vi "Agilent 2000 3000 X-Series Control Loop Response Analysis.vi"() -> ()   [LabVIEW 2015]
doc: "This example shows how to apply a control loop response analysis and read the analysis result."
uses:
  Agilent 2000 3000 X-Series.lvlib
  Public/Configure/Power Analysis/Configure Control Loop Response Power Analysis (Basic).vi
  Public/Data/Read Control Loop Response Power Analysis (Data).vi
  Public/Configure/Power Analysis/Configure Control Loop Response Power Analysis (Frequency).vi
  Public/Data/Read Control Loop Response Power Analysis (Gain).vi
  Public/Configure/Power Analysis/Configure Control Loop Response Power Analysis (Waveform).vi
panel:
  in  "Stop Frequency (6: 20000000 Hz)":i32(ring)=6 items=["100", "1000", "10000", "100000", "1000000", "10000000", "20000000"]
  in  "Start Frequency (1: 100 Hz)":i32(ring)=1 items=["20", "100", "1000", "10000", "100000", "1000000", "10000000"]
  out "Analysis Result":string[][](table)
  in  "Point Number (10: 10)":i32(ring)=10 items=["10"=10, "20"=20, "30"=30, "40"=40, "50"=50, "60"=60, "70"=70, "80"=80, "90"=90, "100"=100]
  in  "Amplitude (0.2)":dbl=0.2
  in  "VISA resource name":refnum<visa-resource-name>
  out "Phase Crossover Frequency (Hz)":dbl
  out "Gain Margin (dB)":dbl
  in  "Impedance (1: 50 Ohm)":i32(ring)=1 items=["1 MOhm", "50 Ohm"]
  in  "Trace (4: Gain and Phase)":i32(ring)=4 items=["None", "All", "Gain", "Phase", "Gain and Phase"]
  in  "Input Channel (0: Channel 1)":i32(ring) items=["Channel 1", "Channel 2", "Channel 3", "Channel 4"]
  in  "Output Channel (1: Channel 2)":i32(ring)=1 items=["Channel 1", "Channel 2", "Channel 3", "Channel 4"]
  # "(c) 2018 - 2023 National Instruments.  ALL RIGHTS RESERVED."
  # "Control Loop Response Analysis settings"
  # "Result"
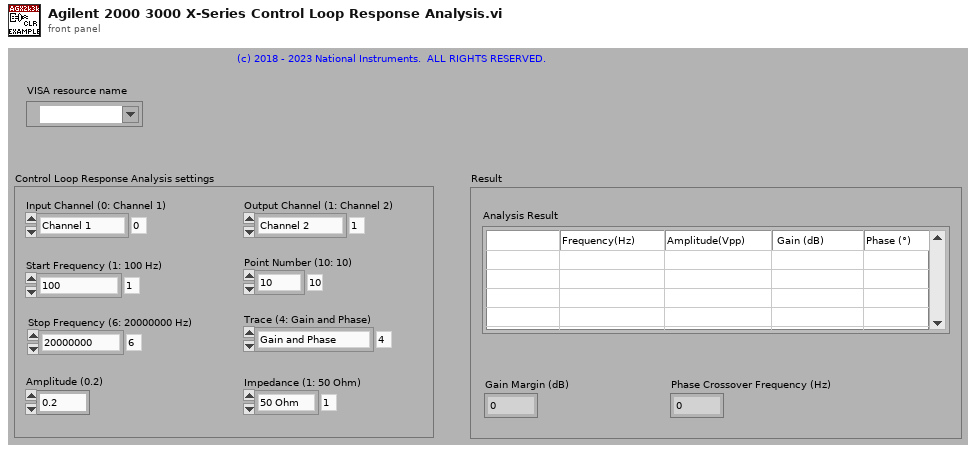
[diagram p1: front panel]
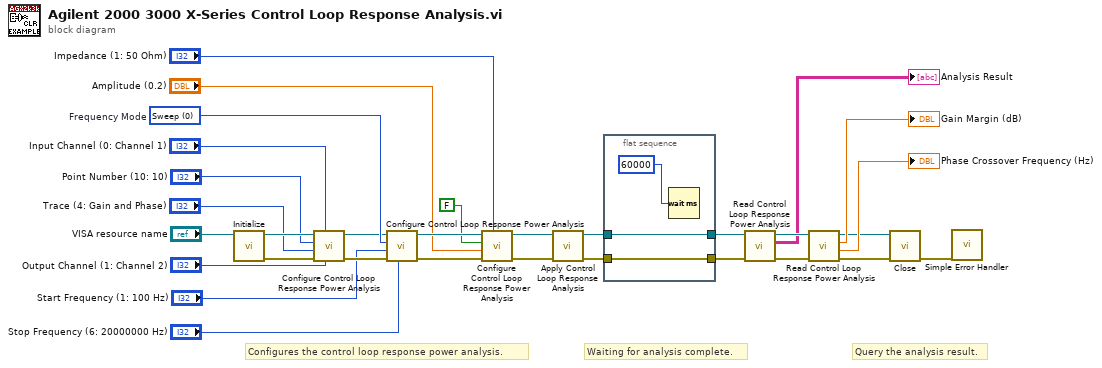
[diagram p0: block diagram]
diagram:
  w31 = 0 items=["Sweep", "Single"]  # Frequency Mode
  # "Query the analysis result."
  # "Waiting for analysis complete."
  # "Configures the control loop response power analysis."
  n1 = call "Initialize.vi"("VISA resource name"="VISA resource name") -> ("error out"=w22:errorcluster, "VISA resource name out"=w23:refnum<visa-resource-name>)  [unwired: 4 in, 5 out]
  n2 = call-poly "Configure Control Loop Response Power Analysis.vi"("Output Channel (1: Channel 2)"="Output Channel (1: Channel 2)", "Input Channel (0: Channel 1)"="Input Channel (0: Channel 1)", "error in (no error)"=w22, "Trace (4: Gain and Phase)"="Trace (4: Gain and Phase)", "Point Number (10: 10)"="Point Number (10: 10)", "VISA resource name"=w23) -> ("error out"=w19:errorcluster, "VISA resource name out"=w27:refnum<visa-resource-name>)  [unwired: 4 in]
  n3 = call-poly "Configure Control Loop Response Power Analysis.vi"("Stop Frequency (6: 20000000 Hz)"="Stop Frequency (6: 20000000 Hz)", "error in (no error)"=w19, "Start Frequency (1: 100 Hz)"="Start Frequency (1: 100 Hz)", "Frequency Mode (0: Sweep)"=w31, "VISA resource name"=w27) -> ("error out"=w18:errorcluster, "VISA resource name out"=w26:refnum<visa-resource-name>)  [unwired: 5 in]
  n4 = call-poly "Configure Control Loop Response Power Analysis.vi"("Impedance (1: 50 Ohm)"="Impedance (1: 50 Ohm)", "error in (no error)"=w18, "Amplitude (0.2)"="Amplitude (0.2)", "Enable Initial Ramp Amplitude (F: Disable)"=FALSE ("Enable Initial Ramp Amplitude (T: Enable)"), "VISA resource name"=w26) -> ("error out"=w8:errorcluster, "VISA resource name out"=w10:refnum<visa-resource-name>)  [unwired: 5 in]
  n5 = call "Apply Control Loop Response Analysis.vi"("error in (no error)"=w8, "VISA resource name"=w10) -> ("error out"=w7:errorcluster, "VISA resource name out"=w9:refnum<visa-resource-name>)  [unwired: 8 in]
  n6 = flat-sequence {
    tunnel: w9 -> [w33]
    tunnel: w7 -> [w32]
    tunnel: [w33] -> w6
    tunnel: [w32] -> w5
    frame #0 {
      n7 = Wait (ms)(milliseconds to wait=60000) -> ()  [unwired: 1 out]
    }
  }
  n8 = call-poly "Read Control Loop Response Power Analysis.vi"("error in (no error)"=w5, "VISA resource name"=w6) -> ("error out"=w17:errorcluster, "Analysis Result"=→"Analysis Result":string[][], "VISA resource name out"=w25:refnum<visa-resource-name>)  [unwired: 7 in]
  n9 = call-poly "Read Control Loop Response Power Analysis.vi"("error in (no error)"=w17, "VISA resource name"=w25) -> ("error out"=w16:errorcluster, "Phase Crossover Frequency (Hz)"=→"Phase Crossover Frequency (Hz)":dbl, "Gain Margin (dB)"=→"Gain Margin (dB)":dbl, "VISA resource name out"=w21:refnum<visa-resource-name>)  [unwired: 6 in]
  n10 = call "Close.vi"("error in (no error)"=w16, "VISA resource name"=w21) -> ("error out"=w20:errorcluster)  [unwired: 9 out]
  n11 = call <vilib>:"Simple Error Handler.vi"("error in (no error)"=w20) -> ()  [unwired: 1 in, 8 out]
